vi "Serial data.vi"(8 "error in":errorcluster, 10 "Serial Number":string, 11 "refnum in":refnum<file>) -> (0 "error out":errorcluster, 3 "refnum out":refnum<file>)   [LabVIEW 2018]
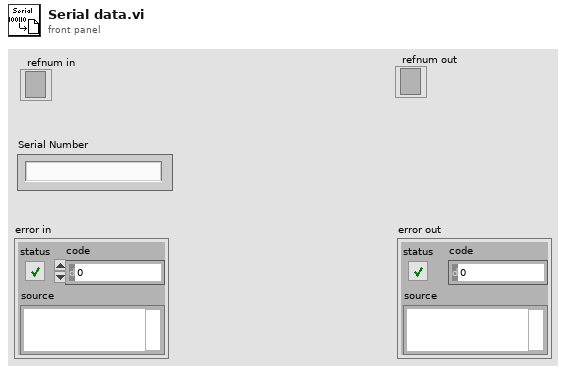
[diagram p1: front panel]
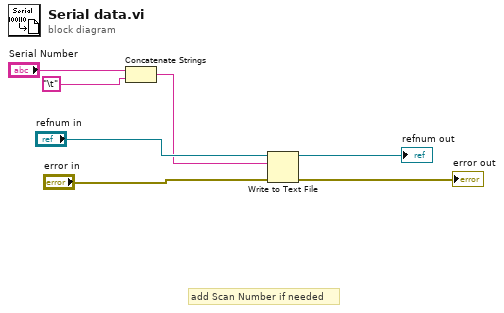
[diagram p0: block diagram]
diagram:
  # "add Scan Number if needed"
  n1 = Concatenate Strings("Serial Number", "\t") -> (w3:string)
  n2 = Write to Text File(file (use dialog)="refnum in", text=w3, error in="error in") -> (refnum out=→"refnum out":refnum<file>, error out=→"error out":errorcluster)  [unwired: 1 in, 1 out]
